vi "Demo - Read Digital Inputs Continuously.vi"() -> ()   [LabVIEW 2021]
uses:
  TypeDefs/Enum - Machine State.ctl
  TypeDefs/TypeDef - Cluster of DAQiFi Device Properties.ctl
  TypeDefs/Enum - Connection Type.ctl
  <vilib>/ErrorRing/Error Ring.xnode
panel:
  out "Digital Inputs":bool[](array[boolean])
  in  "Stop":bool
  in  "DAQ IP or COM":string="192.168.1.1"
  # "0     1     2     3     4     5     6     7     8     9    10   11   12   13   14   15"
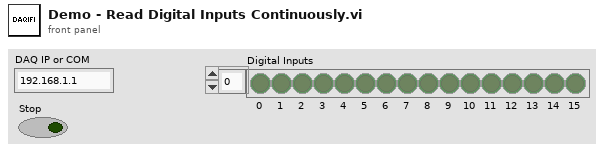
[diagram p1: front panel]
types:
  T1 = typedef "TypeDef - Cluster of DAQiFi Device Properties.ctl" = cluster{"IP Address":string, "MAC Address":string, "Serial Number":string, "Connection Type":T2, "Connected":bool, "TCP Network Connection":refnum<k5>, "USB Serial Connection":refnum<visa-resource-name>}
  T2 = typedef "Enum - Connection Type.ctl" = enum16{"USB", "TCP"}
  T3 = typedef "Enum - Machine State.ctl" = enum16{"Shutdown", "Save Data", "Start Streaming", "Initialize", "Read Streamed Data"}
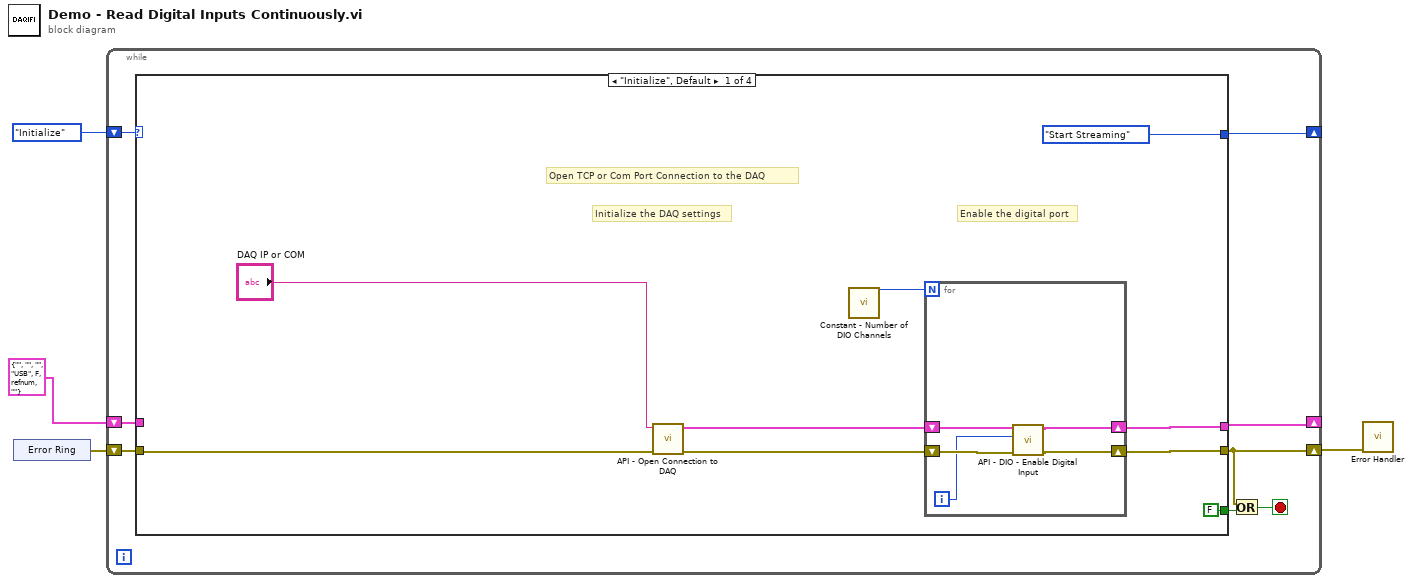
[diagram p0: block diagram]
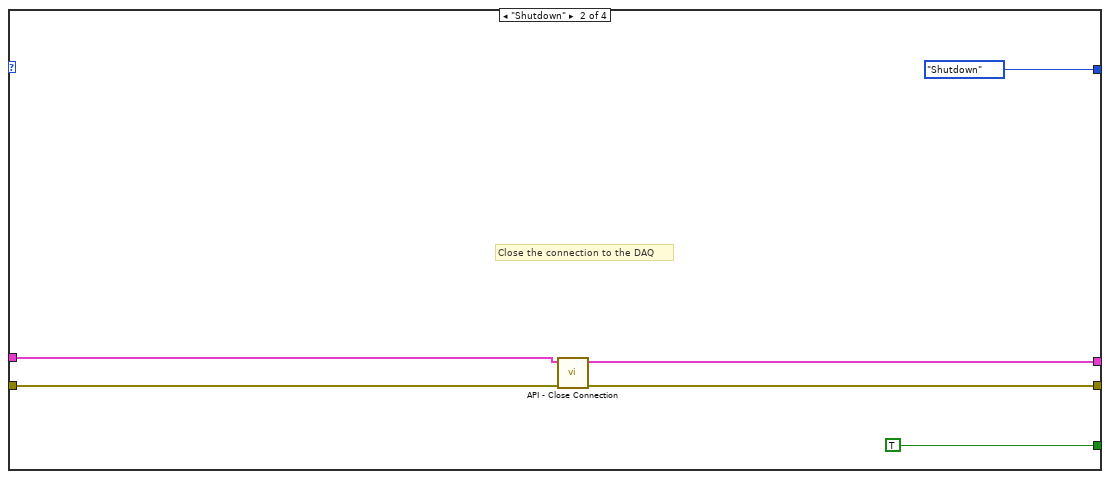
[diagram p2: hidden frame]
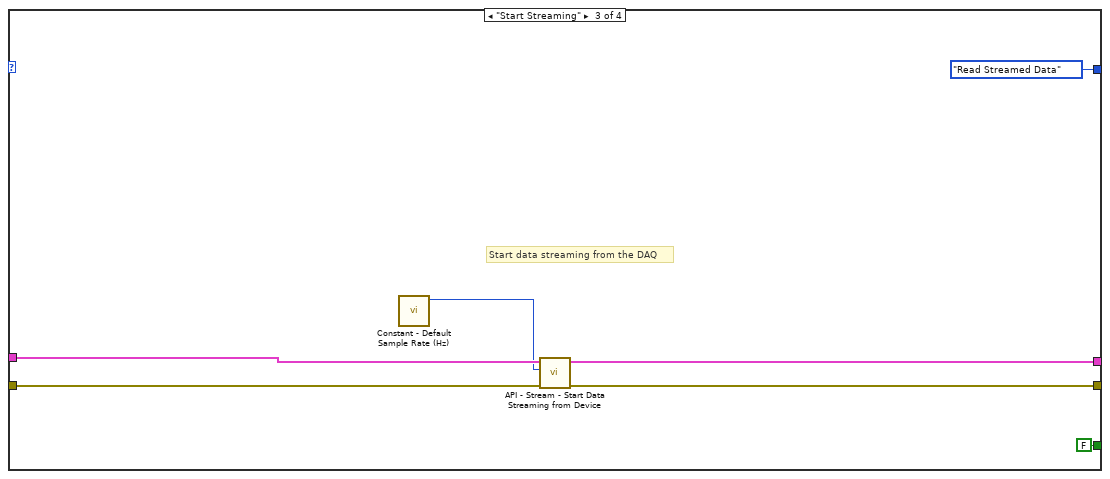
[diagram p3: hidden frame]
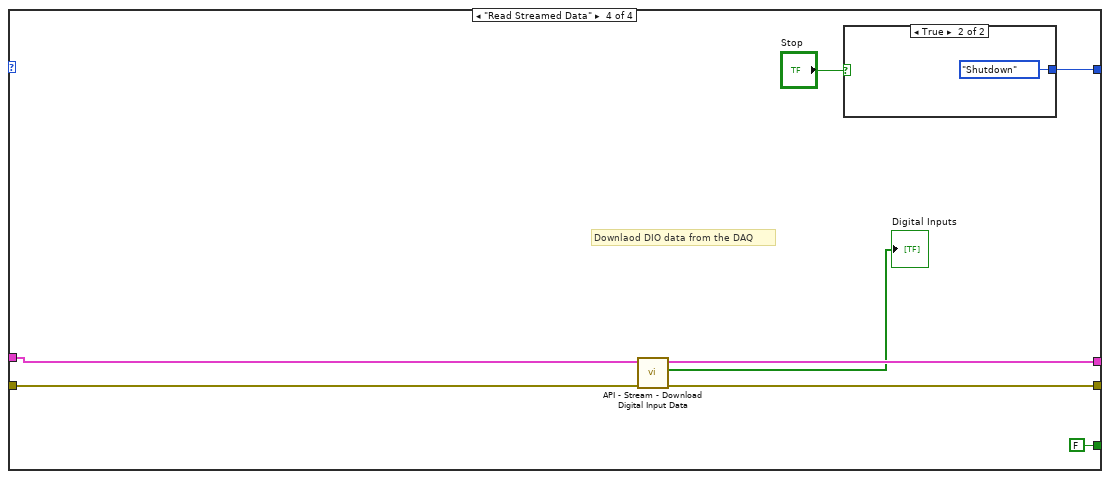
[diagram p4: hidden frame]
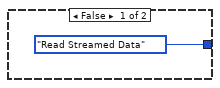
[diagram p5: hidden frame]
diagram:
  n1 = xnode "Error Ring"() -> ("error out"=w3:errorcluster)
  n2 = while {
    shift-right: [w6] -> w2
    shift-left: w3 -> [w11]
    shift-right: [w10] -> _
    shift-left: T1 {"IP Address"="", "MAC Address"="", "Serial Number"="", "Connection Type"=enum."USB", "Connected"=FALSE, "TCP Network Connection"=refnum, "USB Serial Connection"=""} ("DAQiFi Device Properties Out") -> [w8]
    shift-right: [w9] -> _
    shift-left: Enum_-_Machine_State."Initialize" -> [w12]
    stop <- w5 stop-if-true
    n3 = case shown="\"Initialize\", Default" w12 {
      tunnel: w11 -> [w14 w29 w35 w43]
      tunnel: [w19 w28 w34 w44] -> w6
      tunnel: [w18 w27 w37 w45] -> w10
      tunnel: [Enum_-_Machine_State."Start Streaming" Enum_-_Machine_State."Shutdown" Enum_-_Machine_State."Read Streamed Data" w47] -> w9
      tunnel: [FALSE TRUE FALSE FALSE] -> w7
      tunnel: w8 -> [_ w30 w36 w46]
      frame "Initialize", Default {
        # "Enable the digital port"
        # "Open TCP or Com Port Connection to the DAQ"
        # "Initialize the DAQ settings"
        n4 = call "API - Open Connection to DAQ.vi"("error in"=w14, "DAQ Address (IP or COM)"="DAQ IP or COM") -> ("error out"=w13:errorcluster, "DAQiFi Device Properties"=w16:T1)  [unwired: 8 in]
        n5 = call "Constant - Number of DIO Channels.vi"() -> ("Maximum Channel"=w17:i32)  [unwired: 11 in]
        n6 = for {
          N: w17 -> [_]
          shift-right: [w23] -> w18
          shift-left: w16 -> [w26]
          shift-right: [w24] -> w19
          shift-left: w13 -> [w25]
          i -> [w22]
          n7 = call "API - DIO - Enable Digital Input.vi"("error in"=w25, "Channel Number"=w22, "DAQiFi Device Properties In"=w26) -> ("error out"=w24:errorcluster, "DAQiFi Device Properties Out"=w23:T1)  [unwired: 7 in]
        }
      }
      frame "Shutdown" {
        # "Close the connection to the DAQ"
        n8 = call "API - Close Connection.vi"("error in"=w29, "DAQiFi Device Properties In"=w30) -> ("error out"=w28:errorcluster, "DAQiFi Device Properties Out"=w27:T1)  [unwired: 8 in]
      }
      frame "Start Streaming" {
        # "Start data streaming from the DAQ"
        n9 = call "Constant - Default Sample Rate (Hz).vi"() -> ("Streaming Rate (Hz)"=w33:i32)  [unwired: 11 in]
        n10 = call "API - Stream - Start Data Streaming from Device.vi"("error in"=w35, "Streaming Rate (Hz)"=w33, "DAQiFi Device Properties In"=w36) -> ("error out"=w34:errorcluster, "DAQiFi Device Properties Out"=w37:T1)  [unwired: 7 in]
      }
      frame "Read Streamed Data" {
        # "Downlaod DIO data from the DAQ"
        n11 = call "API - Stream - Download Digital Input Data.vi"("error in"=w43, "DAQiFi Device Properties In"=w46) -> ("error out"=w44:errorcluster, "Digital Inputs"=→"Digital Inputs":bool[], "DAQiFi Device Properties Out"=w45:T1)  [unwired: 7 in]
        n12 = case shown="True" "Stop" {
          tunnel: [Enum_-_Machine_State."Read Streamed Data" Enum_-_Machine_State."Shutdown"] -> w47
          frame False {
          }
          frame True {
          }
        }
      }
    }
    n13 = Or(x=w6, y=w7) -> (x .or. y?=w5:bool)
  }
  n14 = call "Error Handler.vi"("error in"=w2) -> ()  [unwired: 10 in, 1 out]
